vi "PXIe-4130_Initialize.vi"(0 "Instrument Info":T1, 1 "User Reference":i32, 5 "error in (no error)":errorcluster) -> (19 "error out":errorcluster)   [LabVIEW 2018, in "PXIe-4130.lvclass"]
uses:
  PXIe-4130.lvclass
  Station/Station Support/Controls/Instrument Info.ctl
  C:/Users/John Gmitter/OneDrive - National Instruments/Git Repo/Harris-FL/Reference Management Server/Instrument Drivers/Power_Supply/Power_Supply Virtual/Power_Supply Virtual.lvclass
  PXIe-4130.lvclass/PXIe-4130.ctl
  Power_Supply Virtual/Power_Supply Virtual.lvclass
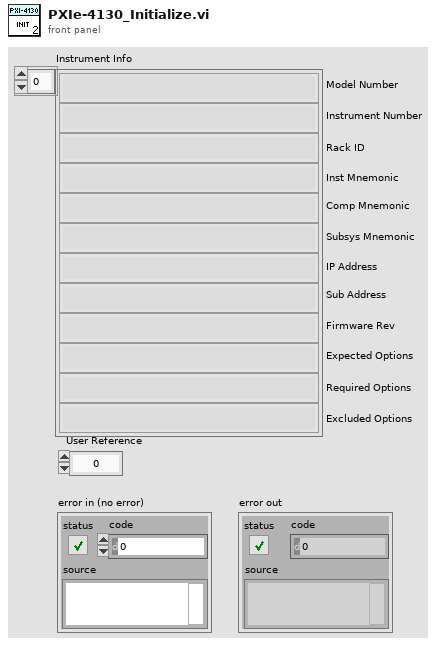
[diagram p1: front panel]
types:
  T1 = typedef "Instrument Info.ctl" = string[]
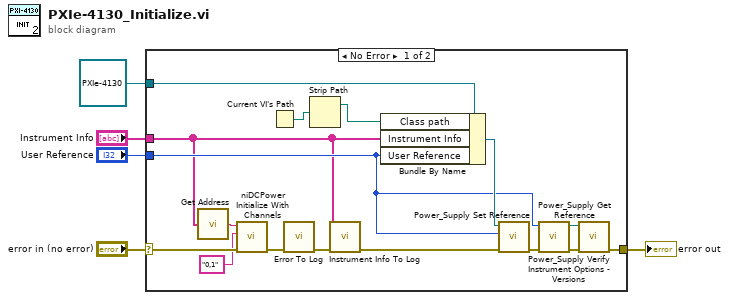
[diagram p0: block diagram]
diagram:
  n1 = case shown="No Error" "error in (no error)" {
    selector: "error in (no error)" -> [w12 w22]
    tunnel: [w17 w22] -> w4
    tunnel: "Instrument Info" -> [w9 _]
    tunnel: "User Reference" -> [w19 _]
    tunnel: refnum<class "PXIe-4130.lvclass"> refnum ("PXIe-4130.lvclass") -> [w13 _]
    frame No Error {
      n2 = call "Get Address.vi"("Instrument Info"=w9) -> ("Address"=w10:string)  [unwired: 4 in]
      n3 = call <instrlib>:"niDCPower Initialize With Channels.vi"("error in (no error)"=w12, "channels"="0,1", "resource name"=w10) -> ("error out"=w11:errorcluster)  [unwired: 7 in, 1 out]
      n4 = Current VI's Path() -> (path=w7:path)
      n5 = call "Error To Log.vi"("error in (no error)"=w11) -> ("error out"=w14:errorcluster)  [unwired: 14 in]
      n6 = Strip Path(path=w7) -> (stripped path=w6:path)  [unwired: 1 out]
      n7 = call "Instrument Info To Log.vi"("Instrument Info"=w9, "error in (no error)"=w14) -> ("error out"=w15:errorcluster)  [unwired: 13 in]
      n8 = Bundle By Name(cluster=w13, "Class path"=w6, "Instrument Info"=w9, "User Reference"=w19) -> (w21:refnum<class "PXIe-4130.lvclass">)
      n9 = call "Power_Supply Set Reference.vi"("error in (no error)"=w15, "User Reference"=w19, "Power_Supply Virtual.lvclass"=w21) -> ("error out"=w20:errorcluster)  [unwired: 8 in]
      n10 = call "Power_Supply Get Reference.vi"("error in (no error)"=w20, "Instrument Reference"=w19) -> ("error out"=w18:errorcluster, "Power_Supply Virtual.lvclass"=w16:refnum<class "Power_Supply Virtual.lvclass">)  [unwired: 7 in, 1 out]
      n11 = call-dynamic "Power_Supply Verify Instrument Options - Versions.vi"("error in (no error)"=w18, "Power_Supply Virtual in"=w16) -> ("error out"=w17:errorcluster)  [unwired: 8 in, 1 out]
    }
    frame Error {
    }
  }
  "error out" <- w4
